vi "wriotefileWithoutInitiate.vi"() -> ()   [LabVIEW 2015]
panel:
  in  "file (use dialog)":path
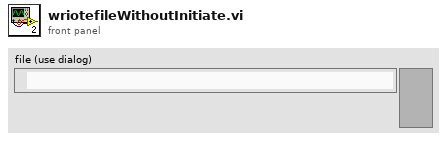
[diagram p1: front panel]
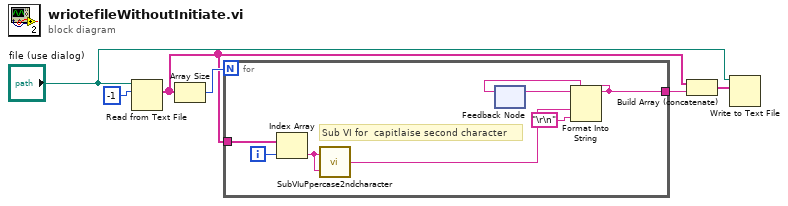
[diagram p0: block diagram]
diagram:
  n1 = Read from Text File(file (use dialog)="file (use dialog)", count=-1) -> (text=w3:string[])  [unwired: 2 in, 3 out]
  n2 = Array Size(array=w3) -> (size(s)=w5:i32)
  n3 = for {
    N: w5 -> [_]
    tunnel: w3 -> [w13]
    tunnel: [w8] -> w2
    i -> [w11]
    # "Sub VI for  capitlaise second character"
    n4 = Index Array(array=w13, index=w11) -> (element=w12:string)
    n5 = call "SubVIuPpercase2ndcharacter.vi"("substring"=w12, "string"=w12) -> ("result string"=w10:string)
    n6 = feedback #1() -> (w7:string)  [unwired: 1 in]
    n7 = Format Into String(initial string=w7, w10, "\r\n") -> (resulting string=w8:string)  [unwired: 2 in, 1 out]
    n8 = feedback-in #1(w8) -> ()
  }
  n9 = Build Array (concatenate)(w3, w2) -> (w1:string[])
  n10 = Write to Text File(file (use dialog)="file (use dialog)", text=w1) -> ()  [unwired: 2 in, 3 out]
